vi "enumerateStaticDependencies.vi"(8 "error in (no error)":errorcluster, 11 "SMO":refnum<class "SMO.lvclass">) -> (0 "error out":errorcluster, 2 "Static Dependencies":refnum<class "Dependency.lvclass">[](array[class]), 3 "SMO out":refnum<class "SMO.lvclass">)   [LabVIEW 2013, in "SMO.lvclass"]
uses:
  SMO.lvclass
  Dependency/Dependency.lvclass
panel:
  # "For instructions on how to use the JKI State Machine Objects, examples and video tutorials, visit:\nhttp://jki.net/state-machine-objects/\n\nJKI State Machine Objects™\nhttp://jki.net/state-machine-objects/\nCopyright (C) 2005-2015, JKI <info@jki.net>\nALL RIGHTS RESERVED"
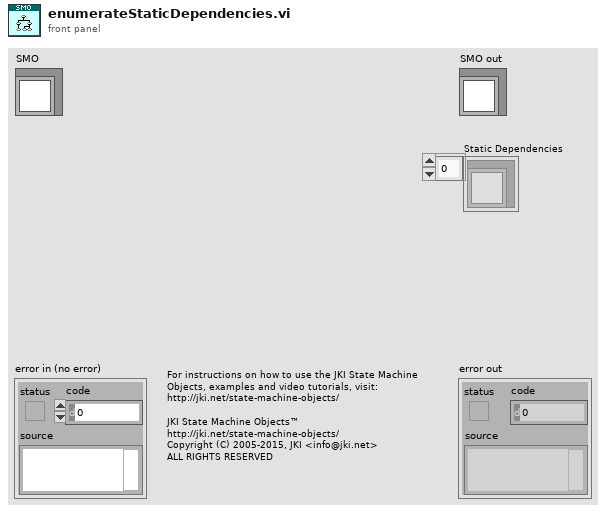
[diagram p1: front panel]
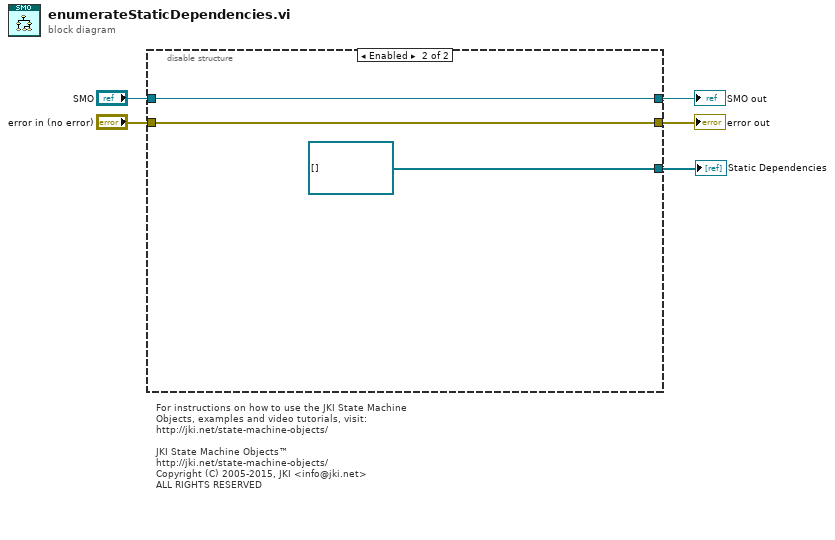
[diagram p0: block diagram]
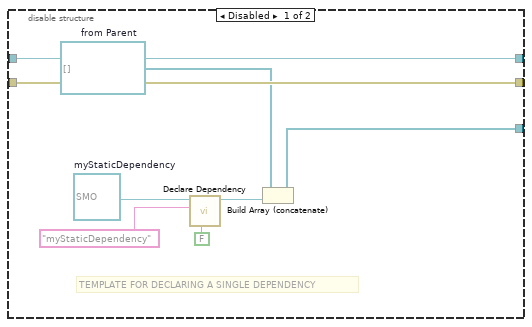
[diagram p2: hidden frame]
diagram:
  # "For instructions on how to use the JKI State Machine Objects, examples and video tutorials, visit:\nhttp://jki.net/state-machine-objects/\n\nJKI State Machine Objects™\nhttp://jki.net/state-machine-objects/\nCopyright (C) 2005-2015, JKI <info@jki.net>\nALL RIGHTS RESERVED"
  n1 = disable-structure shown="Enabled" {
    disable-tunnel: "SMO" -> [w13 w16]
    disable-tunnel: [w13 w16] -> w4
    disable-tunnel: "error in (no error)" -> [w12 w15]
    disable-tunnel: [w12 w15] -> w2
    disable-tunnel: [w7 refnum<class "Dependency.lvclass">[] [] ("appended array")] -> w1
    frame Disabled {
      w6 = refnum<class "Dependency.lvclass">[] []  # from Parent
      w11 = refnum<class "SMO.lvclass"> refnum  # myStaticDependency
      # "TEMPLATE FOR DECLARING A SINGLE DEPENDENCY"
      n2 = call "Declare Dependency.vi"("Shared Resource (F)"=FALSE, "Name"="myStaticDependency", "Type"=w11) -> ("Dependency out"=w8:refnum<class "Dependency.lvclass">)  [unwired: 7 in, 1 out]
      n3 = Build Array (concatenate)(w6, w8) -> (w7:refnum<class "Dependency.lvclass">[])
    }
    frame Enabled {
    }
  }
  "error out" <- w2
  "SMO out" <- w4
  "Static Dependencies" <- w1
